vi "Run All Jitter Tests Reentrancy_Pretest.vi"(9 "Run in UI?":bool, 10 "Log Path":path, 11 "Jitter Test Folder":path) -> (3 "Total Pass?":bool)   [LabVIEW 2009]
uses:
  VI Reentrancy Setting.ctl
panel:
  in  "Tab Control":enum32{"Instructions", "Test Suite"}(tab)
  in  "Results":string[][](table)
  out "Current Test":string
  out "Current Test Status?":bool
  out "Total Tests":i32
  out "Current Test #":i32
  # "This test analyzes the 'code under investigation' frame of the Jitter Test template\n1) Reentrant settings \n2) Preferred Execution System settings on a VI\nThis applies to all VIs called from the 'code under investigation' and its hierarchy\n\nManual Setup Instructions:\n1) Open a new project and save it\n2) Add this VI to the My Computer Target\n3) Add a RT-Target to the project. If you are using a previously saved project,\n    make sure that the RT-Target has no items added to it, because test suite\n    will first remove these items automatically.\n4) Under the 'Test Suite' tab for this VI, set up the 'Jitter Test Folder' to point to\n    the top-level folder that contains all your jitter tests\n5) Set the 'Log Path' to an xml file record the results of the Test Suite.\n    This is required field\n6) Set 'Run in UI?' to be true\n7) Run the test suite\n\nHow to interpret the 'Results' Table:\n1) 'Results' lists all the VIs in the hierarchy that are currently been analyzed and\n    its status\n2) To check the status of your individual test, you need to look at the log file."
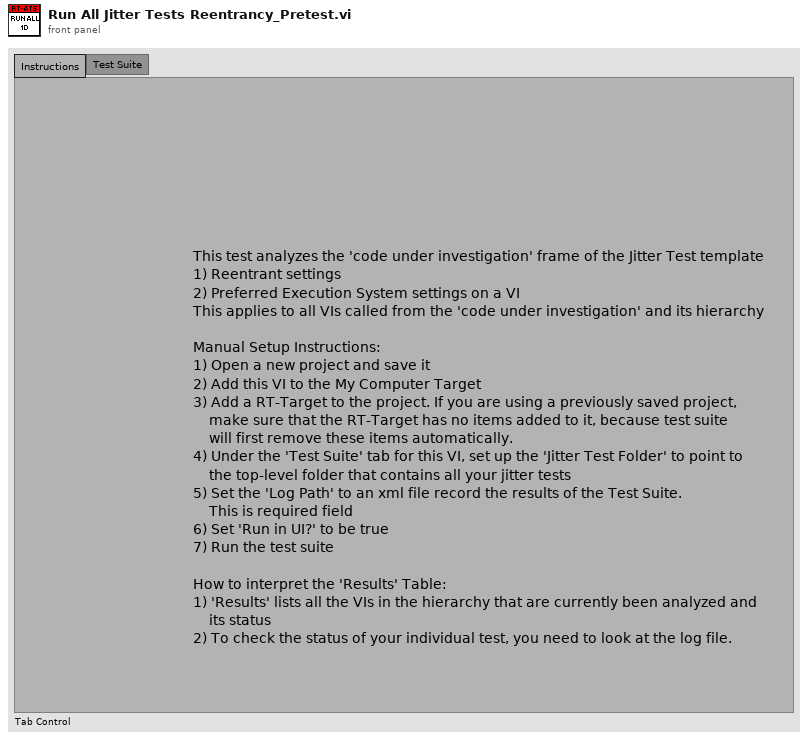
[diagram p1: front panel]
types:
  T1 = enum16{"open", "replace", "create", "open or create", "replace or create", "replace or create with confirmation"}
  T2 = typedef "VI Reentrancy Setting.ctl" = cluster{"VI Name":string, "Path":path, "Reentrant":bool, "Execution:Reentrancy Type":enum16{"Share clones between instances", "Preallocate clone for each instance"}, "Execution:Preferred Exec System":enum32{"invalid execution system", "user interface", "standard", "instrument i/o", "data acquisition", "other 1", "other 2", "same as caller"}, "Exec.Priority":enum32{"invalid priority", "background priority", "normal priority", "above normal priority", "high priority", "time critical priority", "subroutine"}}
  T3 = enum32{"invalid execution system", "user interface", "standard", "instrument i/o", "data acquisition", "other 1", "other 2", "same as caller"}
  T4 = enum32{"invalid priority", "background priority", "normal priority", "above normal priority", "high priority", "time critical priority", "subroutine"}
  T5 = enum16{"Share clones between instances", "Preallocate clone for each instance"}
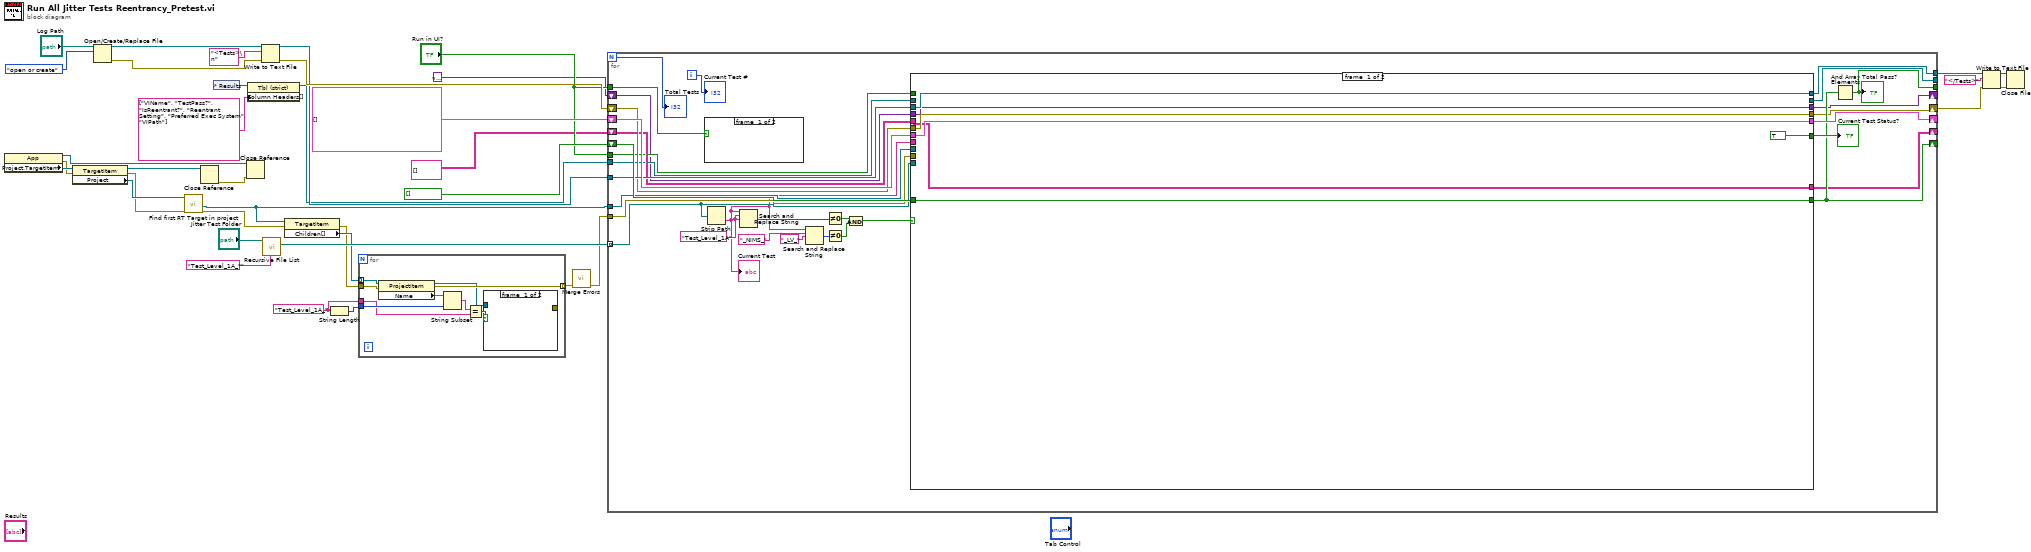
[diagram p0: block diagram]
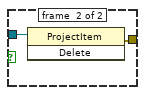
[diagram p2: hidden frame]
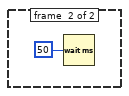
[diagram p3: hidden frame]
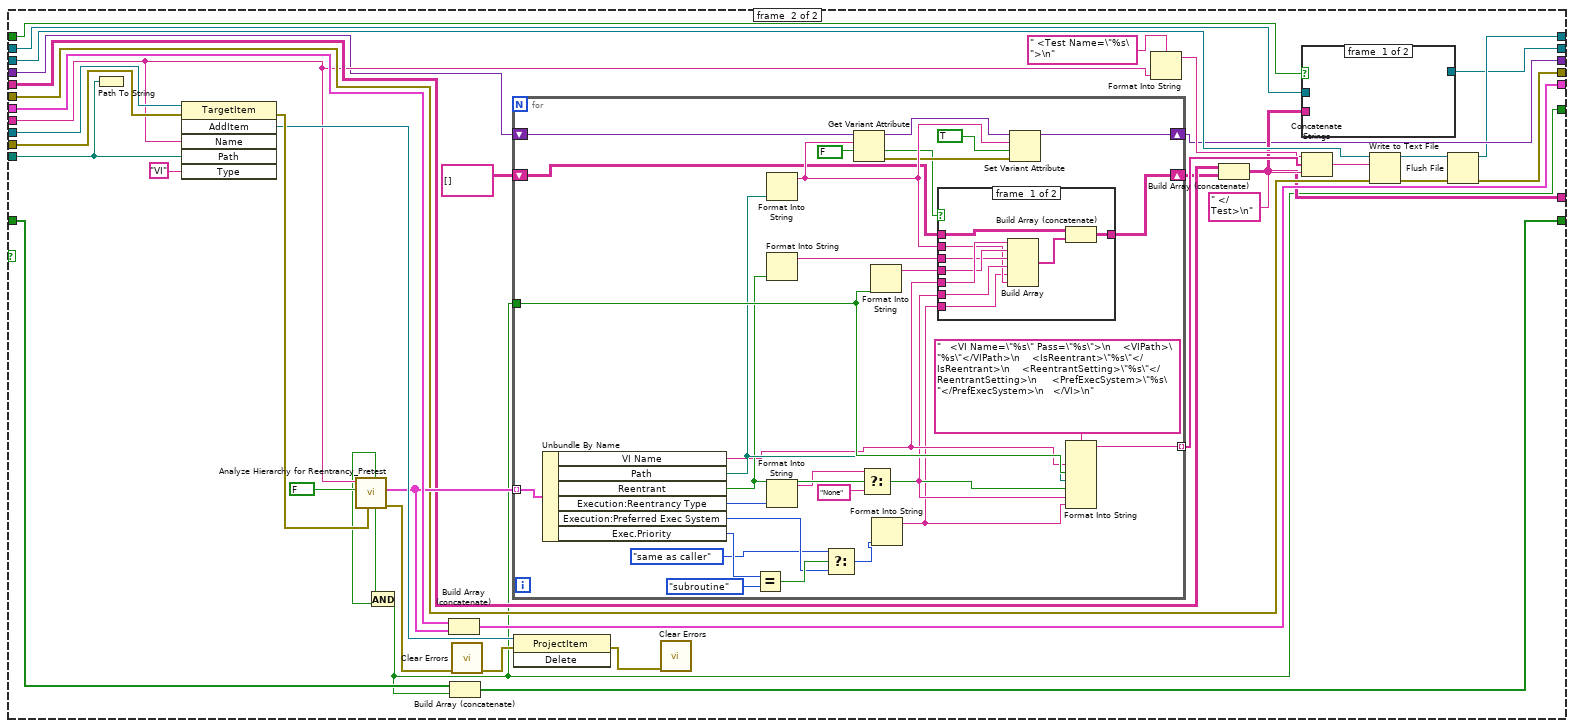
[diagram p4: hidden frame]
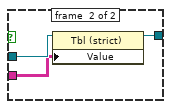
[diagram p5: hidden frame]
diagram:
  w1 = "Test_Level_1A_" ("pattern")
  n1 = property class="App"() -> (reference out=w33:refnum<vi>, error out=w35:errorcluster, "Project.TargetItem"=w38:refnum<vi>)  [unwired: 2 in]
  n2 = property class="TargetItem"(reference=w38, error in=w35) -> (reference out=w30:refnum<vi>, error out=w36:errorcluster, "Project"=w37:refnum<vi>)
  n3 = Open/Create/Replace File(file path (use dialog)="Log Path", operation (0:open)=T1."open or create") -> (refnum out=w21:refnum<file>, error out=w20:errorcluster)  [unwired: 4 in, 1 out]
  n4 = call "Find first RT Target in project.vi"("error in"=w36, "Project Refnum"=w37) -> ("error out"=w29:errorcluster, "Target"=w28:refnum<vi>)  [unwired: 6 in, 2 out]
  n5 = Close Reference(reference=w30) -> (error out=w34:errorcluster)  [unwired: 1 in]
  n6 = control-ref of="Results"() -> (w7:refnum<vi>)
  n7 = Close Reference(reference=w33, error in (no error)=w34) -> ()  [unwired: 1 out]
  n8 = property class="Tbl (strict)"(reference=w7, "Column Headers[]"=string[] ["VIName", "TestPass?", "IsReentrant?", "Reentrant Setting", "Preferred Exec System", "VIPath"] ("Column Header Strings[]")) -> (reference out=w13:refnum<vi>)  [unwired: 1 in, 1 out]
  n9 = Write to Text File(file (use dialog)=w21, text="<Tests>\n", error in=w20) -> (refnum out=w18:refnum<file>, error out=w19:errorcluster)  [unwired: 1 in, 1 out]
  n10 = call <vilib>:"Recursive File List.vi"("pattern"="Test_Level_1A_*", "Folder Path"="Jitter Test Folder") -> ("All Files in Dir"=w27:path[])  [unwired: 5 in, 4 out]
  n11 = property class="TargetItem"(reference=w28, error in=w29) -> (error out=w5:errorcluster, "Children[]"=w6:refnum<vi>[])  [unwired: 1 out]
  n12 = String Length(string=w1) -> (length=w2:i32)
  n13 = for {
    tunnel: w6 -> [w47] mode=indexing
    tunnel: w5 -> [w46]
    tunnel: [w45] -> w4 mode=indexing
    tunnel: w2 -> [w43]
    tunnel: w1 -> [w41]
    n14 = property class="ProjectItem"(reference=w47, error in=w46) -> (reference out=w39:refnum<vi>, error out=w45:errorcluster, "Name"=w44:string)
    n15 = String Subset(string=w44, length (rest)=w43) -> (substring=w42:string)  [unwired: 1 in]
    n16 = Equal?(x=w42, y=w41) -> (x = y?=w40:bool)
    n17 = case shown="True" w40 {
      tunnel: w39 -> [_ w49]
      tunnel: [_ w48] -> _
      frame #0 {
      }
      frame #1 {
        n18 = invoke class="ProjectItem" method="Delete"(reference=w49) -> (error out=w48:errorcluster)  [unwired: 2 in, 2 out]
      }
    }
  }
  n19 = call <vilib>:"Merge Errors.vi"("error array in"=w4) -> ("error out"=w3:errorcluster)  [unwired: 6 in]
  n20 = for {
    N -> [w80]
    shift-right: [w69] -> _
    shift-left: T2[] [] ("Array") -> [w72]
    shift-right: [w68] -> _
    shift-left: bool[] [] -> [w70]
    tunnel: w27 -> [w66] mode=indexing
    tunnel: w28 -> [w67]
    tunnel: w3 -> [w65]
    tunnel: w18 -> [w62]
    tunnel: [w61] -> w24
    shift-right: [w60] -> w8
    shift-left: w19 -> [w59]
    tunnel: [w58] -> _
    shift-right: [w57] -> _
    shift-left: string[][] [] -> [w56]
    tunnel: w13 -> [w55]
    tunnel: "Run in UI?" -> [w54]
    tunnel: "Run in UI?" -> [w53]
    shift-right: [w51] -> _
    shift-left: variant ("variant") -> [w52]
    tunnel: [w50] -> _
    i -> [w81]
    w79 = "Test_Level_1A"
    n21 = case shown="True" w54 {
      frame #0 {
      }
      frame #1 {
        n22 = Wait (ms)(milliseconds to wait=u32 50) -> ()  [unwired: 1 out]
      }
    }
    n23 = Strip Path(path=w66) -> (name=w64:string)  [unwired: 1 out]
    "Current Test" <- w64
    n24 = Search and Replace String(input string=w64, search string=w79, replace string=w79) -> (number of replacements=w76:i32)  [unwired: 5 in, 3 out]
    n25 = Search and Replace String(input string=w64, search string="_NIMS_", replace string="_LV_") -> (number of replacements=w75:i32)  [unwired: 5 in, 3 out]
    n26 = Not Equal To 0?(x=w76) -> (x != 0?=w73:bool)
    n27 = Not Equal To 0?(x=w75) -> (x != 0?=w74:bool)
    n28 = And(x=w73, y=w74) -> (x .and. y?=w63:bool)
    n29 = case shown="True" w63 {
      tunnel: [w88 w125] -> w68
      tunnel: [w89 w126] -> w69
      tunnel: w72 -> [w89 w127]
      tunnel: [TRUE ("Worked?") w91] -> w71
      tunnel: w70 -> [w88 w124]
      tunnel: w67 -> [_ w123]
      tunnel: w66 -> [_ w103]
      tunnel: w65 -> [_ w121]
      tunnel: w64 -> [_ w104]
      tunnel: w62 -> [w86 w113]
      tunnel: w59 -> [w85 w111]
      tunnel: [w86 w96] -> w61
      tunnel: [w85 w98] -> w60
      tunnel: [w84 w107] -> w57
      tunnel: w56 -> [w84 w109]
      tunnel: w55 -> [_ w110]
      tunnel: w53 -> [_ w90]
      tunnel: w52 -> [w83 w102]
      tunnel: [w83 w100] -> w51
      tunnel: [_ w95] -> w50
      frame #0 {
      }
      frame #1 {
        n30 = Path To String(path=w103) -> ()  [unwired: 1 out]
        n31 = invoke class="TargetItem" method="AddItem"(reference=w123, error in=w121, "Name"=w104, "Path"=w103, "Type"="VI") -> (error out=w120:errorcluster, "AddItem"=w119:refnum<vi>)  [unwired: 1 in, 4 out]
        n32 = call "Analyze Hierarchy for Reentrancy_Pretest.vi"("error in (no error)"=w120, "Require Preallocated Reentrancy"=FALSE, "Test Name"=w104) -> ("error out"=w106:errorcluster, "Array"=w117:T2[], "Reentrancy OK?"=w93:bool, "Preferred Exec System OK?"=w92:bool)  [unwired: 3 in, 2 out]
        n33 = And(x=w93, y=w92) -> (x .and. y?=w91:bool)
        n34 = Build Array (concatenate)(w127, w117) -> (w126:T2[])
        n35 = Build Array (concatenate)(w124, w91) -> (w125:bool[])
        n36 = call <vilib>:"Clear Errors.vi"("error in (no error)"=w106) -> ("error out"=w105:errorcluster)  [unwired: 6 in]
        n37 = for {
          tunnel: w117 -> [w161] mode=indexing
          tunnel: [w159] -> w116 mode=indexing
          tunnel: w91 -> [w157]
          shift-right: [w139] -> w108
          shift-left: string[][] [] -> [w142]
          shift-right: [w140] -> w100
          shift-left: w102 -> [w146]
          n38 = Unbundle By Name(w161) -> ("VI Name"=w154:string, "Path"=w156:path, "Reentrant"=w155:bool, "Execution:Reentrancy Type"=w158:T5, "Execution:Preferred Exec System"=w134:T3, "Exec.Priority"=w137:T4)
          n39 = Equal?(x=w137, y=T4."subroutine") -> (x = y?=w135:bool)
          n40 = Format Into String(w156) -> (resulting string=w144:string)  [unwired: 3 in, 1 out]
          n41 = Format Into String(w155) -> (resulting string=w152:string)  [unwired: 3 in, 1 out]
          n42 = Format Into String(w158) -> (resulting string=w150:string)  [unwired: 3 in, 1 out]
          n43 = Select(t=T3."same as caller", s=w135, f=w134) -> (s? t:f=w133:T3)
          n44 = Get Variant Attribute(Variant=w146, name=w144, default value (empty Variant)=FALSE) -> (duplicate Variant=w145:variant, value=w141:bool, error out=w143:errorcluster)  [unwired: 1 in, 1 out]
          n45 = Select(t=w150, s=w155, f="None" ("t")) -> (s? t:f=w151:string)
          n46 = Format Into String(w157) -> (resulting string=w153:string)  [unwired: 3 in, 1 out]
          n47 = Format Into String(w133) -> (resulting string=w138:string)  [unwired: 3 in, 1 out]
          n48 = case shown="True" w141 {
            tunnel: w154 -> [w170 _]
            tunnel: w153 -> [w169 _]
            tunnel: w152 -> [w168 _]
            tunnel: w151 -> [w167 _]
            tunnel: [w163 w171] -> w139
            tunnel: w144 -> [w166 _]
            tunnel: w142 -> [w165 w171]
            tunnel: w138 -> [w162 _]
            frame #0 {
              n49 = Build Array(w170, w169, w168, w167, w162, w166) -> (w164:string[])
              n50 = Build Array (concatenate)(w165, w164) -> (w163:string[][])
            }
            frame #1 {
            }
          }
          n51 = Set Variant Attribute(Variant=w145, name=w144, value=TRUE, error in=w143) -> (Variant out=w140:variant)  [unwired: 2 out]
          n52 = Format Into String(format string="   <VI Name=\"%s\" Pass=\"%s\">\n    <VIPath>\"%s\"</VIPath>\n    <IsReentrant>\"%s\"</IsReentrant>\n    <ReentrantSetting>\"%s\"</ReentrantSetting>\n     <PrefExecSystem>\"%s\"</PrefExecSystem>\n   </VI>\n", w154, w157, w156, w155, w151, w138) -> (resulting string=w159:string)  [unwired: 2 in, 1 out]
        }
        n53 = invoke class="ProjectItem" method="Delete"(reference=w119, error in=w105) -> (error out=w94:errorcluster)  [unwired: 1 in, 2 out]
        n54 = call <vilib>:"Clear Errors.vi"("error in (no error)"=w94) -> ()  [unwired: 6 in, 1 out]
        n55 = Format Into String(format string=" <Test Name=\"%s\">\n", w104) -> (resulting string=w115:string)  [unwired: 2 in, 1 out]
        n56 = Build Array (concatenate)(w109, w108) -> (w107:string[][])
        n57 = case shown="True" w90 {
          tunnel: w110 -> [_ w131]
          tunnel: w107 -> [_ w130]
          tunnel: [_ w129] -> w95
          frame #0 {
          }
          frame #1 {
            n58 = property class="Tbl (strict)"(reference=w131, "Value"=w130) -> (reference out=w129:refnum<vi>)  [unwired: 1 in, 1 out]
          }
        }
        n59 = Concatenate Strings(w115, w116, " </Test>\n") -> (w112:string)
        n60 = Write to Text File(file (use dialog)=w113, text=w112, error in=w111) -> (refnum out=w97:refnum<file>, error out=w99:errorcluster)  [unwired: 1 in, 1 out]
        n61 = Flush File(refnum=w97, error in=w99) -> (refnum out=w96:refnum<file>, error out=w98:errorcluster)
      }
    }
    "Current Test Status?" <- w71
    n62 = And Array Elements(Boolean array=w68) -> (logical AND=w58:bool)
    "Total Pass?" <- w58
    "Current Test #" <- w81
    "Total Tests" <- w80
  }
  n63 = Write to Text File(file (use dialog)=w24, text="</Tests>", error in=w8) -> (refnum out=w22:refnum<file>, error out=w23:errorcluster)  [unwired: 1 in, 1 out]
  n64 = Close File(refnum=w22, error in=w23) -> ()  [unwired: 2 out]
